vi "Select Splitter.vi"(8 "error in (no error)":errorcluster, 10 "Pane Index":i32, 11 "This VI":refnum<vi>) -> (0 "error out":errorcluster, 2 "Splitter":refnum<vi>, 3 "Pane":refnum<vi>)   [LabVIEW 2014]
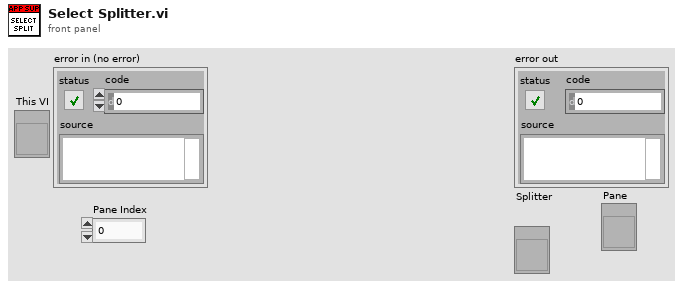
[diagram p1: front panel]
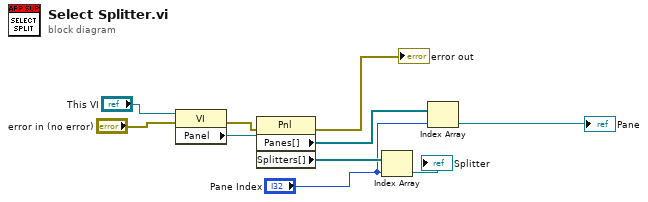
[diagram p0: block diagram]
diagram:
  n1 = property class="VI"(reference="This VI", error in="error in (no error)") -> (error out=w7:errorcluster, "Panel"=w8:refnum<vi>)  [unwired: 1 out]
  n2 = property class="Pnl"(reference=w8, error in=w7) -> (error out=→"error out":errorcluster, "Panes[]"=w3:refnum<vi>[], "Splitters[]"=w6:refnum<vi>[])  [unwired: 1 out]
  n3 = Index Array(array=w6, index="Pane Index") -> (element=→"Splitter":refnum<vi>)
  n4 = Index Array(array=w3, index="Pane Index") -> (element=→"Pane":refnum<vi>)
